vi "Find Structure ID from DFT ID.vi"(8 "error in (no error)":errorcluster, 10 "DFT ID":string, 11 "connection reference":T1) -> (0 "error out":errorcluster, 1 "POSCAR ID":string, 2 "CONTCAR_ID":string, 3 "connection reference out":T1)   [LabVIEW 2010]
uses:
  <vilib>/addons/database/Connection.llb/Conn ObjectReference.ctl
  <vilib>/addons/database/_DB Variant To Data/Database Variant To Data.xnode
  <vilib>/addons/database/NI_Database_API.lvlib
panel:
  out "data":variant[][](array[variant])
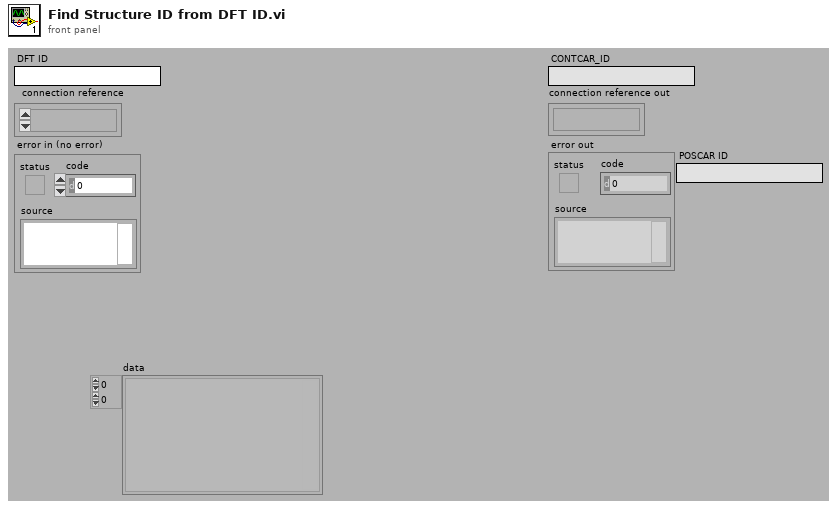
[diagram p1: front panel]
types:
  T1 = typedef "NI_Database_API.lvlib/Conn ObjectReference.ctl" = refnum<k1>
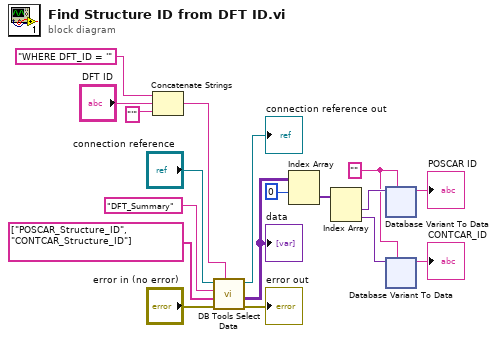
[diagram p0: block diagram]
diagram:
  w4 = ""
  n1 = Concatenate Strings("WHERE DFT_ID = '" ("string"), "DFT ID", "'" ("string")) -> (w13:string)
  n2 = call <vilib>:"DB Tools Select Data.vi"("condition"=w13, "error in (no error)"="error in (no error)", "columns"=string[] ["POSCAR_Structure_ID", "CONTCAR_Structure_ID"], "table"="DFT_Summary", "connection reference"="connection reference") -> ("error out"=→"error out":errorcluster, "data"=w12:variant[][], "connection reference out"=→"connection reference out":T1)  [unwired: 1 in]
  "data" <- w12
  n3 = Index Array(array=w12, index (row)=0) -> (element=w7:variant[])  [unwired: 1 in]
  n4 = Index Array(array=w7) -> (element #1=w6:variant, element #2=w5:variant)  [unwired: 2 in]
  n5 = xnode "Database Variant To Data"("database variant"=w6, "type"=w4) -> ("data"=→"POSCAR ID":string)  [unwired: 1 in, 1 out]
  n6 = xnode "Database Variant To Data"("database variant"=w5, "type"=w4) -> ("data"=→"CONTCAR_ID":string)  [unwired: 1 in, 1 out]
